vi "modbus-to-real.vi"(8 "error in (no error)":errorcluster, 11 "object in":refnum<class "Type-K-Thermocouple.lvclass">) -> (0 "error out":errorcluster, 3 "object out":refnum<class "Type-K-Thermocouple.lvclass">)   [LabVIEW 2021, in "Type-K-Thermocouple.lvclass"]
doc: "Uses adam formula to convert sensors to real No"
uses:
  Type-K-Thermocouple.lvclass
panel:
  # "Conversion of Modbus Reg to a \nType T thermocouple in Degree C"
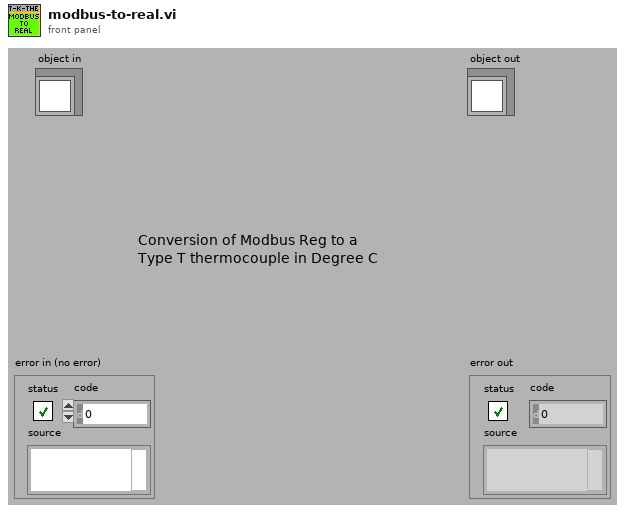
[diagram p1: front panel]
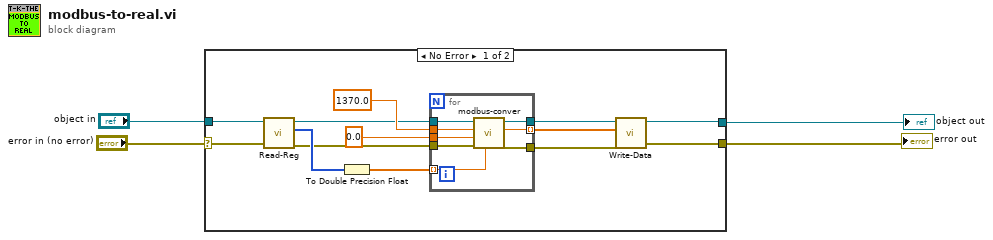
[diagram p0: block diagram]
diagram:
  n1 = case shown="No Error" "error in (no error)" {
    selector: "error in (no error)" -> [w7 w27]
    tunnel: [w13 w27] -> w3
    tunnel: [w15 w26] -> w1
    tunnel: "object in" -> [w12 w26]
    frame No Error {
      n2 = call-dynamic "Read-Reg.vi"("error in (no error)"=w7, "Type-K-Thermocouple in"=w12) -> ("error out"=w6:errorcluster, "Modbus-Reg"=w11:u16[], "Type-K-Thermocouple out"=w9:refnum<class "Type-K-Thermocouple.lvclass">)  [unwired: 7 in]
      n3 = To Double Precision Float(number=w11) -> (double precision float=w10:dbl[])
      n4 = for {
        tunnel: w9 -> [w25]
        tunnel: 1370.0 ("Scale Max Range") -> [w23]
        tunnel: 0.0 ("Scale Min range") -> [w22]
        tunnel: [w24] -> w5
        tunnel: [w21] -> w14 mode=indexing
        tunnel: w10 -> [w20] mode=indexing
        tunnel: [w19] -> w8
        tunnel: w6 -> [w18]
        n5 = call-dynamic "modbus-conver.vi"("Reg"=w20, "error in (no error)"=w18, "Scale Min range"=w22, "Scale Max Range"=w23, "object in"=w25) -> ("error out"=w24:errorcluster, "output"=w21:dbl, "object out"=w19:refnum<class "Type-K-Thermocouple.lvclass">)  [unwired: 4 in]
      }
      n6 = call-dynamic "Write-Data.vi"("error in (no error)"=w5, "Data"=w14, "Type-K-Thermocouple in"=w8) -> ("error out"=w13:errorcluster, "Type-K-Thermocouple out"=w15:refnum<class "Type-K-Thermocouple.lvclass">)  [unwired: 7 in]
    }
    frame Error {
    }
  }
  "error out" <- w3
  "object out" <- w1
